vi "APS get task info.vi"(8 "error in (no error)":errorcluster caption="错误输入（无错误）", 9 "Info":T1, 10 "TaskNum":i32, 11 "Board_ID":i32) -> (0 "error out":errorcluster caption="错误输出", 1 "Info out":T1, 3 "function return":i32)   [LabVIEW 2011, in "APS168.lvlib"]
doc: "I32 FNTYPE APS_get_task_info( I32 Board_ID, I32 TaskNum, TSK_INFO *Info );"
uses:
  APS168.lvlib
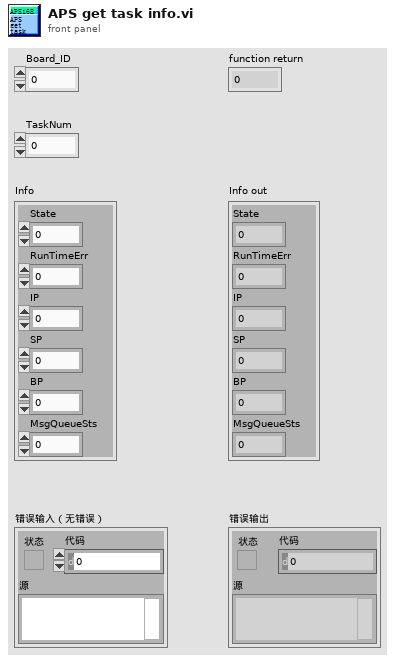
[diagram p1: front panel]
types:
  T1 = cluster{"State":u16, "RunTimeErr":u16, "IP":u16, "SP":u16, "BP":u16, "MsgQueueSts":u16}
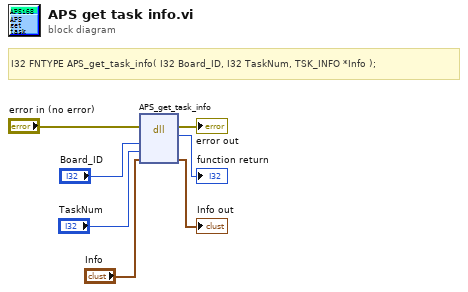
[diagram p0: block diagram]
diagram:
  # "I32 FNTYPE APS_get_task_info( I32 Board_ID, I32 TaskNum, TSK_INFO *Info );"
  n1 = dll-call lib="PTH1Labs E软件ADLINK 204CAPS_1_7_1_LIB line 连续运动204APS168.*" fn="APS_get_task_info"(error in="error in (no error)", "Board_ID"="Board_ID", "TaskNum"="TaskNum", "Info"="Info") -> (error out=→"error out":errorcluster, →"function return":i32, "Info"=→"Info out":T1)  [unwired: 4 in, 1 out]
